vi "rs485trials.vi"() -> ()   [LabVIEW 2019]
uses:
  Desktop/Thesis/LabVIEW/Simple Serial With Time delays in between for each byte/support/Serial - Settings.ctl
  <vilib>/Instr/_visa.llb/VISA Configure Serial Port (Instr).vi
panel:
  out "read buffer":string
  in  "Scaling 2":dbl=10000000000.0 format="%#_13g"
  out "Real RPM":string
  out "realrpm":dbl(graph)
  in  "byte order (0:big-endian, network order) 2":T1(ring)=enum."little-endian"
  out "message":string="Error -1073807194 occurred at Property Node (arg 8) in VISA Configure Serial Port (Instr).vi->rs485trials.vi\r\n\r\nPossible reason(s):\n\r\nVISA:  (Hex 0xBFFF00A6) The connection for the given session has been lost."
  in  "Esrar":string="\u0002\u0003IX\u0000\u0002S·"
  in  "stop":bool
  in  "VISA resource name":refnum<visa-resource-name>="COM1"
  in  "Serial Settings":T2={"baud rate"=19200, "data bits"=8, "parity"=enum."Even", "stop bits"=10, "flow control"=0} {"flow control" items=["None"=0, "XON/XOFF"=1, "RTS/CTS"=2, "DTR/DSR"=4]; "stop bits" items=["1.0"=10, "1.5"=15, "2.0"=20]; "data bits" min=5 max=8 step=1; "baud rate" items=["75"=75, "110"=110, "134"=134, "150"=150, "300"=300, "600"=600, "1200"=1200, "1800"=1800, "2400"=2400, "4800"=4800, "7200"=7200, "19600"=9600, "14400"=14400, "19200"=19200, "28800"=28800, "38400"=38400, "56000"=56000, "57600"=57600, "115200"=115200, "128000"=128000, "230400"=230400]}
  out "Serial Settings:Wire Mode":i8(ring)=-128 items=["Unknown"=-1, "RS485/Wire4"=0, "RS485/Wire2-EchoDTR"=1, "RS485/Wire2-CtrlDTR"=2, "RS485/Wire2-Auto"=3, "RS232/DTE"=-128, "RS232/DCE"=-127, "RS232/Auto"=-126]
  in  "Enable Termination\nChar (T)":bool
  in  "timeout (10sec)":u32=10000
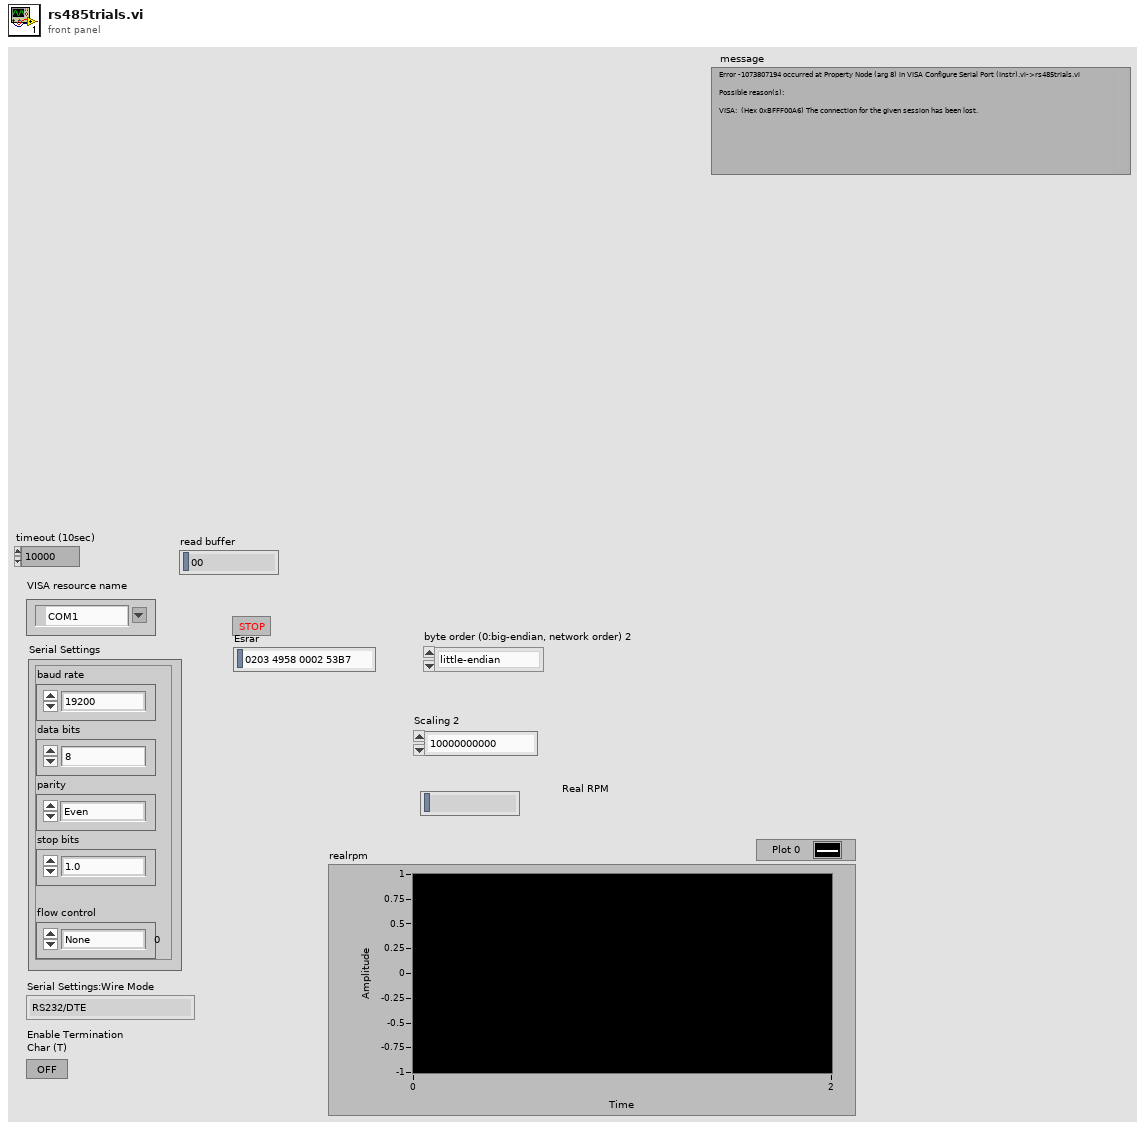
[diagram p1: front panel]
types:
  T1 = enum16{"big-endian, network order", "native, host order", "little-endian"}
  T2 = typedef "Serial - Settings.ctl" = cluster{"baud rate":u32, "data bits":u16, "parity":enum16{"None", "Odd", "Even", "Mark", "Space"}, "stop bits":u16, "flow control":u16}
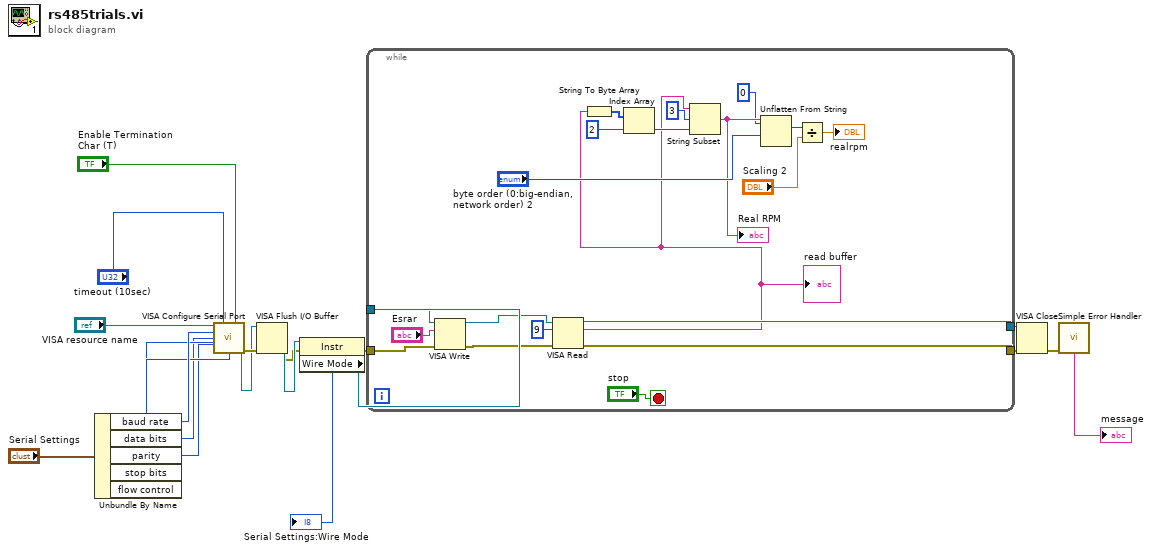
[diagram p0: block diagram]
diagram:
  n1 = Unbundle By Name("Serial Settings") -> ("baud rate"=w13:u32, "data bits"=w9:u16, "parity"=w10:enum16{"None", "Odd", "Even", "Mark", "Space"}, "stop bits"=w11:u16, "flow control"=w12:u16)
  n2 = call-poly "VISA Configure Serial Port"("VISA resource name"="VISA resource name", "timeout (10sec)"="timeout (10sec)", "Enable Termination\nChar (T)"="Enable Termination\nChar (T)", "baud rate (9600)"=w13, "data bits (8)"=w9, "parity (0:none)"=w10, "stop bits (10: 1 bit)"=w11, "flow control (0:none)"=w12) -> ("VISA resource name out"=w18:refnum<visa-resource-name>, "error out"=w19:errorcluster)  [unwired: 1 in, 5 out]
  n3 = VISA Flush I/O Buffer(VISA resource name=w18, error in (no error)=w19) -> (VISA resource name out=w17:refnum<visa-resource-name>, error out=w16:errorcluster)  [unwired: 1 in]
  n4 = property class="Instr"(reference=w17, error in=w16) -> (reference out=w6:refnum<visa-resource-name>, error out=w5:errorcluster, "Wire Mode"=→"Serial Settings:Wire Mode":i16)
  n5 = while {
    tunnel: w6 -> [w39]
    tunnel: w5 -> [w38]
    tunnel: [w34] -> w2
    tunnel: [w33] -> w1
    stop <- "stop" stop-if-true
    n6 = VISA Write(VISA resource name=w39, write buffer="Esrar", error in (no error)=w38) -> (VISA resource name out=w35:refnum<visa-resource-name>, error out=w36:errorcluster)  [unwired: 1 out]
    n7 = VISA Read(VISA resource name=w35, byte count=u32 9, error in (no error)=w36) -> (VISA resource name out=w34:refnum<visa-resource-name>, read buffer=w21:string, error out=w33:errorcluster)  [unwired: 1 out]
    "read buffer" <- w21
    n8 = String To Byte Array(string=w21) -> (unsigned byte array=w30:u8[])
    n9 = Index Array(array=w30, index=2) -> (element=w27:u8)
    n10 = String Subset(string=w21, offset (0)=3, length (rest)=w27) -> (substring=w26:string)
    "Real RPM" <- w26
    n11 = Unflatten From String(type=0, binary string=w26, byte order (0:big-endian, network order)="byte order (0:big-endian, network order) 2") -> (value=w23:i32)  [unwired: 2 in, 2 out]
    n12 = Divide(x=w23, y="Scaling 2") -> (x/y=→"realrpm":dbl)
  }
  n13 = VISA Close(VISA resource name=w2, error in (no error)=w1) -> (error out=w4:errorcluster)
  n14 = call <vilib>:"Simple Error Handler.vi"("error in (no error)"=w4) -> ("message"=→"message":string)  [unwired: 1 in, 7 out]
